vi "Digital - Finite Output.vi"() -> ()   [LabVIEW 2022 SP3]
doc: "This example demonstrates how to generate a finite amount of digital data based off of a sample clock.\n\nSome hardware (e.g. M Series DAQ) must use an external sample clock for digital tasks. To view a complete list of available sample clock sources, consult the Device Routes table in Measurement and Automation Explorer.\n\nFor instructions on how to connect your signals to the DAQ device, refer to your device documentation."
uses:
  <vilib>/Utility/error.llb/DialogType.ctl
  <vilib>/DAQmx/write.llb/DAQmx Write (Digital 1D U32 1Chan NSamp).vi
  <vilib>/DAQmx/create/channels.llb/DAQmx Create Channel (DO-Digital Output).vi
  <vilib>/DAQmx/configure/timing.llb/DAQmx Timing (Sample Clock).vi
  <vilib>/DAQmx/configure/trigger.llb/DAQmx Start Trigger (Digital Edge).vi
  <vilib>/DAQmx/configure/trigger.llb/DAQmx Start Trigger (Time).vi
  <vilib>/DAQmx/miscellaneous.llb/DAQmx Fill In Error Info.vi
  <resource>/objmgr/daqmx.rc
panel:
  in  "Output Array":u32[](array[numeric])=[1, 2, 4, 8, 16, 32, 64, 128]
  in  "Trigger Type":T1(tab)
  in  "Edge":i32(ring)=10280 items=["Rising"=10280, "Falling"=10171]
  in  "Digital Trigger Source":tag="PFI1"
  in  "When":timestamp
  in  "Select Time\nManually":bool
  in  "Number of Samples":i32=1000
  in  "Sample Rate":dbl=1000.0
  in  "Sample Clock Source":tag="PFI0"
  out "Actual Sample Rate":dbl=1000.0 format="%0.2f"
  in  "Line(s)":tag="Dev1/port0/line0:7"
  # "Channel Settings"
  # "Data to Write"
  # "Timing and Buffer Settings"
  # "Trigger Settings"
  # "To configure and use a start trigger you must have the necessary tab selected above.  Not all hardware supports triggering--refer to your device documentation for more info."
  # "If time is not manually set, the task will begin after 10 seconds"
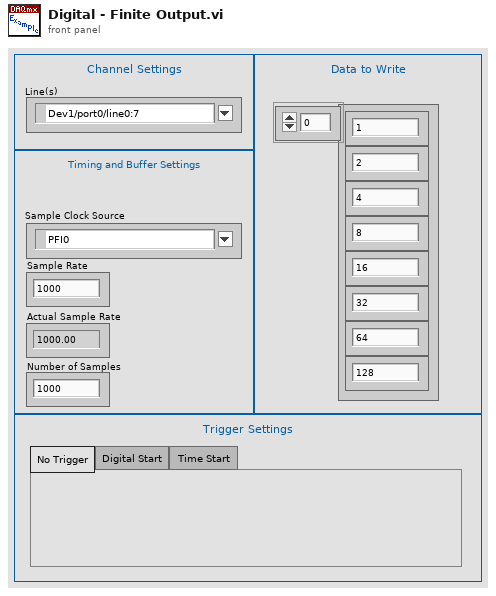
[diagram p1: front panel]
types:
  T1 = enum32{"No Trigger", "Digital Start", "Time Start "}
  T2 = typedef "DialogType.ctl" = u16
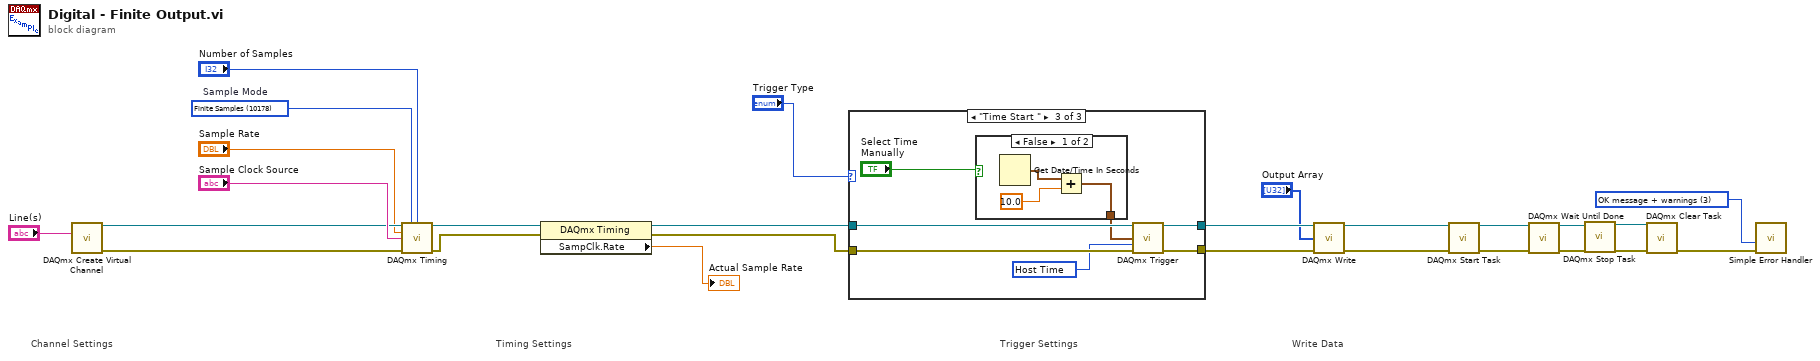
[diagram p0: block diagram]
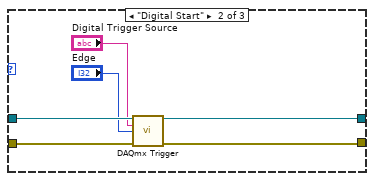
[diagram p3: hidden frame]
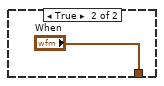
[diagram p4: hidden frame]
diagram:
  w1 = T2 3 items=["no dialog", "OK message", "continue or stop message", "OK message + warnings", "continue/stop + warnings"] ("type of dialog (OK msg:1)")
  w18 = 10178 items=["Finite Samples"=10178, "Continuous Samples"=10123, "Hardware Timed Single Point"=12522]  # Sample Mode
  # "Trigger Settings"
  # "Timing Settings"
  # "Write Data"
  # "Channel Settings"
  n1 = call-poly <vilib>:"DAQmx Create Virtual Channel.vi"("lines"="Line(s)") -> ("task out"=w22:refnum<k21>, "error out"=w21:errorcluster)  [unwired: 13 in]
  n2 = call-poly <vilib>:"DAQmx Timing.vi"("task/channels in"=w22, "sample mode"=w18, "samples per channel"="Number of Samples", "rate"="Sample Rate", "source"="Sample Clock Source", "error in"=w21) -> ("task out"=w17:refnum<k21>, "error out"=w16:errorcluster)  [unwired: 8 in]
  n3 = property class="DAQmx Timing"(reference=w17, error in=w16) -> (reference out=w14:refnum<k21>, error out=w13:errorcluster, "SampClk.Rate"=→"Actual Sample Rate":dbl)
  n4 = case shown="\"Time Start \"" "Trigger Type" {
    tunnel: w14 -> [w28 w34 w41]
    tunnel: w13 -> [w27 w33 w40]
    tunnel: [w28 w32 w39] -> w12
    tunnel: [w27 w31 w38] -> w11
    frame "No Trigger", Default {
    }
    frame "Digital Start" {
      n5 = call-poly <vilib>:"DAQmx Trigger.vi"("task/channels in"=w34, "source"="Digital Trigger Source", "edge"="Edge", "error in"=w33) -> ("task out"=w32:refnum<k21>, "error out"=w31:errorcluster)  [unwired: 10 in]
    }
    frame "Time Start " {
      w35 = 16126 items=["Host Time"=16126, "I/O Device Time"=16127] ("timescale")
      n6 = case shown="False" "Select Time\nManually" {
        tunnel: [w43 "When"] -> w36
        frame False {
          n7 = Get Date/Time In Seconds() -> (seconds since 1Jan1904=w44:timestamp)
          n8 = Add(x=w44, y=10.0) -> (x+y=w43:timestamp)
        }
        frame True {
        }
      }
      n9 = call-poly <vilib>:"DAQmx Trigger.vi"("task/channels in"=w41, "when"=w36, "timescale"=w35, "error in"=w40) -> ("task out"=w39:refnum<k21>, "error out"=w38:errorcluster)  [unwired: 10 in]
    }
  }
  n10 = call-poly <vilib>:"DAQmx Write.vi"("task/channels in"=w12, "data"="Output Array", "error in"=w11) -> ("task out"=w7:refnum<k21>, "error out"=w6:errorcluster)  [unwired: 10 in, 1 out]
  n11 = call <vilib>:"DAQmx Start Task.vi"("task/channels in"=w7, "error in"=w6) -> ("task out"=w9:refnum<k21>, "error out"=w8:errorcluster)  [unwired: 12 in]
  n12 = call <vilib>:"DAQmx Wait Until Done.vi"("task/channels in"=w9, "error in"=w8) -> ("task out"=w5:refnum<k21>, "error out"=w4:errorcluster)  [unwired: 12 in]
  n13 = call <vilib>:"DAQmx Stop Task.vi"("task/channels in"=w5, "error in"=w4) -> ("task out"=w3:refnum<k21>, "error out"=w2:errorcluster)  [unwired: 12 in]
  n14 = call <vilib>:"DAQmx Clear Task.vi"("task in"=w3, "error in"=w2) -> ("error out"=w26:errorcluster)  [unwired: 13 in]
  n15 = call <vilib>:"Simple Error Handler.vi"("type of dialog (OK msg:1)"=w1, "error in (no error)"=w26) -> ()  [unwired: 3 in, 5 out]
